vi "configureWifi.vi"(0 "connection ID":refnum<k5>, 1 "mode":i32, 2 "SSID":string, 3 "psk":string, 5 "error":errorcluster) -> (14 "connection ID out":refnum<k5>, 19 "error out":errorcluster)   [LabVIEW 2016, in "amc_api.lvlib"]
doc: "Changes the WiFi configuration and applies it."
uses:
  amc_api.lvlib
panel:
  out "jsonRespIn":string
  out "JSON-response":string="{\"jsonrpc\":\"2.0\",\"method\":\"\",\"params\":[5,1.245,true,\"name\"],\"id\":\"1\"}"
  out "JSON request":string
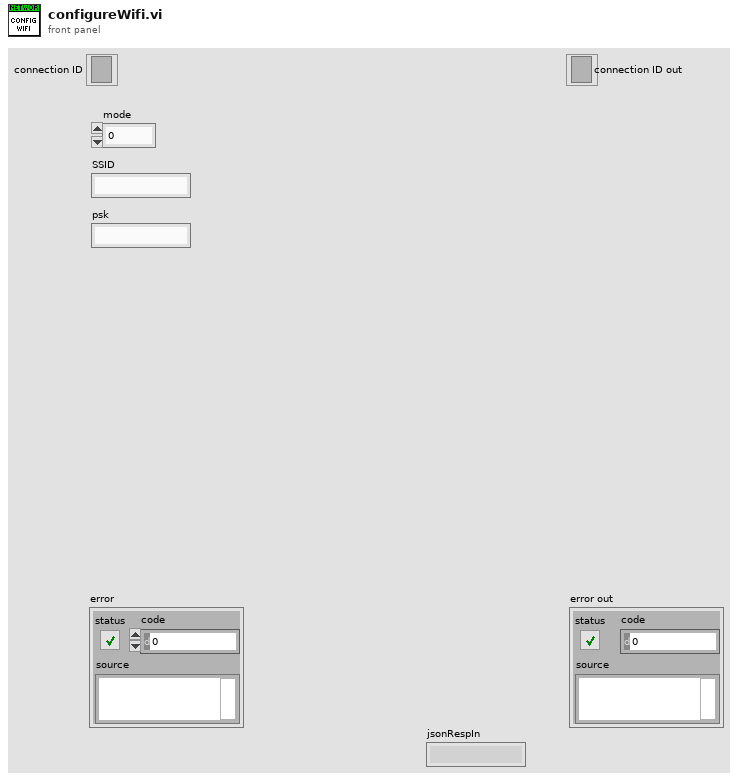
[diagram p1: front panel]
types:
  T1 = cluster{"jsonrpc":string, "method":string, "params":string[], "id":string, "api":i32, "pid":string}
  T2 = enum16{"Standard", "Buffered", "CRLF", "Immediate"}
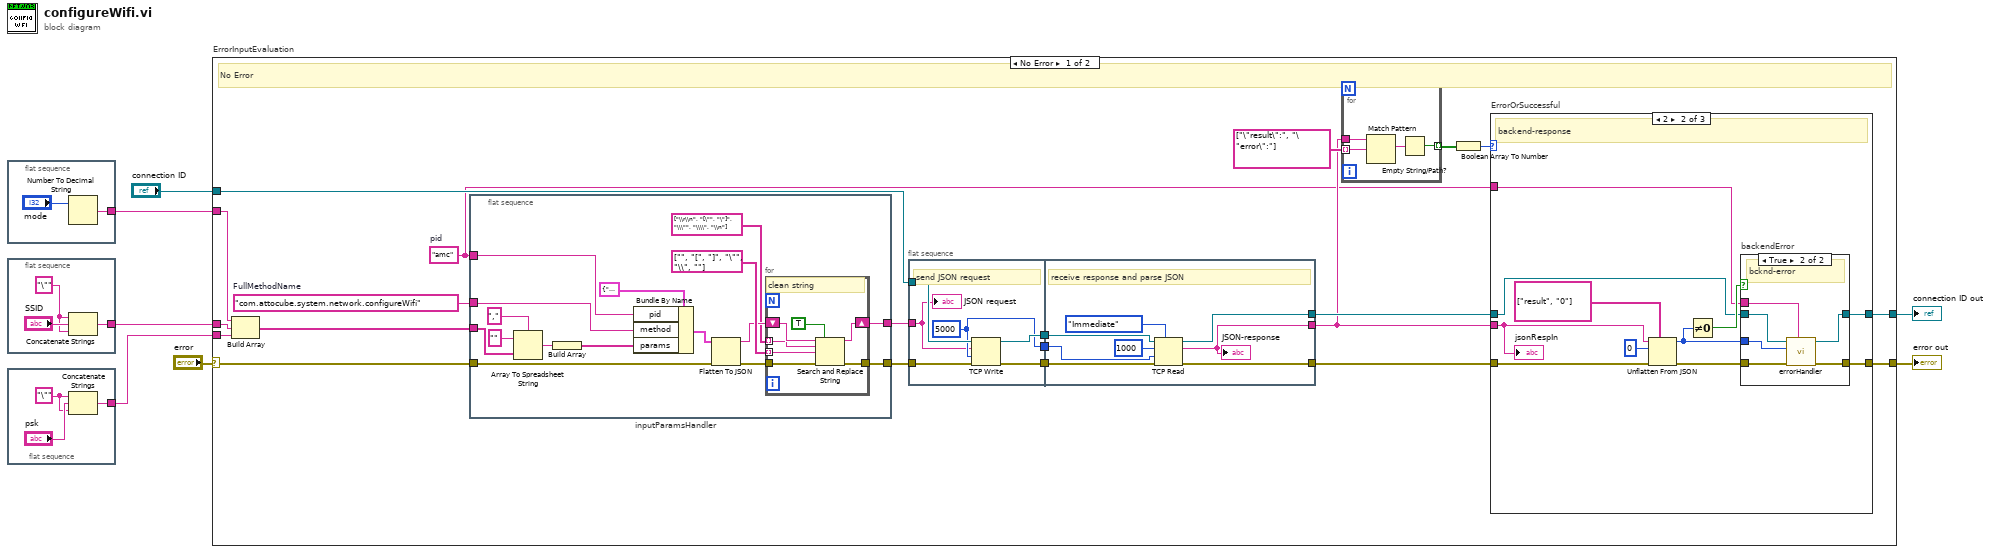
[diagram p0: block diagram]
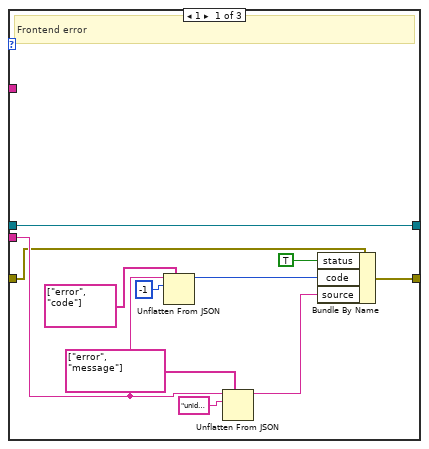
[diagram p2: hidden frame]
diagram:
  n1 = flat-sequence "in_integer" {
    tunnel: [w8] -> w3
    frame #0 {
      n2 = Number To Decimal String(number="mode") -> (decimal integer string=w8:string)  [unwired: 1 in]
    }
  }
  n3 = flat-sequence "in_string" {
    tunnel: [w11] -> w2
    frame #0 {
      w10 = "\"" ("string")
      n4 = Concatenate Strings(w10, "SSID", w10) -> (w11:string)
    }
  }
  n5 = flat-sequence "in_string" {
    tunnel: [w14] -> w1
    frame #0 {
      w13 = "\"" ("string")
      n6 = Concatenate Strings(w13, "psk", w13) -> (w14:string)
    }
  }
  n7 = case "ErrorInputEvaluation" shown="No Error" "error" {
    selector: "error" -> [w29 w110]
    tunnel: "connection ID" -> [w33 w111]
    tunnel: [w20 w110] -> w6
    tunnel: [w21 w111] -> w5
    tunnel: w3 -> [w18 _]
    tunnel: w2 -> [w17 _]
    tunnel: w1 -> [w16 _]
    frame No Error {
      w19 = "amc"  # pid
      w30 = "com.attocube.system.network.configureWifi"  # FullMethodName
      # "No Error"
      n8 = Build Array ("ParametersArrayString")(w18, w17, w16) -> (w28:string[])
      n9 = flat-sequence "inputParamsHandler" {
        tunnel: [w74] -> w27
        tunnel: w28 -> [w80]
        tunnel: w29 -> [w79]
        tunnel: [w76] -> w26
        tunnel: w30 -> [w70]
        tunnel: w19 -> [w69]
        frame #0 {
          n10 = Array To Spreadsheet String(delimiter (Tab)=",", array=w80, 3:"" ("format string")) -> (spreadsheet string=w82:string)
          n11 = Build Array "Build Array"(w82) -> (w71:string[])
          n12 = Bundle By Name(cluster=T1 {"jsonrpc"="2.0", "method"="com.attocube.amc.res.setRESReadOutFreq", "params"=[], "id"="1", "api"=2, "pid"=""} ("Cluster"), "pid"=w69, "method"=w70, "params"=w71) -> (w81:T1)
          n13 = Flatten To JSON(anything=w81, error in (no error)=w79) -> (JSON string=w75:string, 11:w77:errorcluster)  [unwired: 1 in]
          n14 = for {
            tunnel: string[] ["\\r\\n", "[\"", "\"]", "\\\"", "\\\\", "\\n"] ("search string") -> [w88] mode=indexing
            tunnel: string[] ["", "[", "]", "\"", "\\", ""] ("replace string (\"\")") -> [w87] mode=indexing
            shift-right: [w90] -> w74
            shift-left: w75 -> [w89]
            tunnel: w77 -> [w86]
            tunnel: [w85] -> w76
            # "clean string"
            n15 = Search and Replace String(replace all?=TRUE ("replace all? (F)"), input string=w89, search string=w88, replace string=w87, error in=w86) -> (result string=w90:string, error out=w85:errorcluster)  [unwired: 3 in, 2 out]
          }
        }
      }
      n16 = flat-sequence {
        tunnel: w33 -> [w101]
        tunnel: [w99] -> w36
        tunnel: [w100] -> w35
        tunnel: w26 -> [w96]
        tunnel: [w98] -> w34
        tunnel: w27 -> [w97]
        tunnel: [w105] -> w25
        tunnel: w36 -> [w107]
        tunnel: w35 -> [w106]
        tunnel: [w103] -> w24
        tunnel: w34 -> [w104]
        tunnel: [w102] -> w23
        frame #0 {
          w98 = 5000 ("timeout ms (25000)")
          # "send JSON request"
          n17 = TCP Write(connection ID=w101, data in=w97, error in (no error)=w96, 9:w98) -> (connection ID out=w99:refnum<k5>, error out=w100:errorcluster)  [unwired: 1 out]
          "JSON request" <- w97
        }
        frame #1 {
          # "receive response and parse JSON"
          n18 = TCP Read(connection ID=w107, bytes to read=1000, error in (no error)=w106, 7:T2."Immediate" ("mode (standard)"), 9:w104) -> (connection ID out=w105:refnum<k5>, data out=w102:string, error out=w103:errorcluster)
          "JSON-response" <- w102
        }
      }
      n19 = for {
        tunnel: string[] ["\"result\":", "\"error\":"] ("path") -> [w94] mode=indexing
        tunnel: [w92] -> w31 mode=indexing
        tunnel: w23 -> [w95]
        n20 = Match Pattern(string=w95, regular expression=w94) -> (match substring=w93:string)  [unwired: 1 in, 3 out]
        n21 = Empty String/Path?(string/path=w93) -> (empty?=w92:bool)
      }
      n22 = Boolean Array To Number(Boolean array=w31) -> (number=w22:u32)
      n23 = case "ErrorOrSuccessful" shown="2" w22 {
        tunnel: w23 -> [w39 w50 _]
        tunnel: w25 -> [w37 w52 w68]
        tunnel: [w37 w51 w68] -> w21
        tunnel: [w40 w48 w67] -> w20
        tunnel: w24 -> [w38 w49 w67]
        tunnel: w19 -> [_ w53 _]
        frame 1 {
          # "Frontend error"
          n24 = Unflatten From JSON(path=string[] ["error", "code"], JSON string=w39, type and defaults=-1) -> (value=w46:i32)  [unwired: 4 in, 1 out]
          n25 = Unflatten From JSON(path=string[] ["error", "message"], JSON string=w39, type and defaults="unidentified error") -> (value=w47:string)  [unwired: 4 in, 1 out]
          n26 = Bundle By Name(cluster=w38, "status"=TRUE, "code"=w46, "source"=w47) -> (w40:errorcluster)
        }
        frame 2 {
          # "backend-response"
          n27 = Unflatten From JSON(path=string[] ["result", "0"], JSON string=w50, type and defaults=0, error in (no error)=w49) -> (value=w54:i32, error out=w56:errorcluster)  [unwired: 3 in]
          n28 = Not Equal To 0?(x=w54) -> (x != 0?=w55:bool)
          n29 = case "backendError" shown="True" w55 {
            tunnel: w54 -> [_ w66]
            tunnel: w56 -> [w60 w65]
            tunnel: [w59 w64] -> w51
            tunnel: [w60 w63] -> w48
            tunnel: w52 -> [w59 w62]
            tunnel: w53 -> [_ w61]
            frame False {
              # "successful"
            }
            frame True {
              # "bcknd-error"
              n30 = call "errorHandler.vi"("pid"=w61, "error in"=w65, "errNbr"=w66, "connection ID"=w62) -> ("error out 2"=w63:errorcluster, "connection ID out"=w64:refnum<k5>)  [unwired: 6 in]
            }
          }
          "jsonRespIn" <- w50
        }
        frame Default {
          # "NoResponse"
        }
      }
    }
    frame Error {
      # "Error"
    }
  }
  "error out" <- w6
  "connection ID out" <- w5
